vi "New Format.vi"   [LabVIEW 2010]
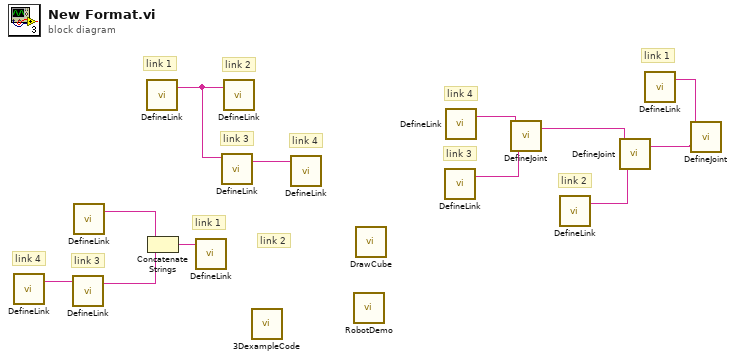
[diagram p0: block diagram]
diagram:
  # "link 1"
  # "link 2"
  # "link 3"
  # "link 4"
  # "link 2"
  # "link 3"
  # "link 4"
  # "link 1"
  # "link 4"
  # "link 3"
  # "link 2"
  # "link 1"
  n1 = call "DefineLink.vi"() -> ("String 2"=w10:string)  [unwired: 4 in]
  n2 = call "DefineLink.vi"("String"=w10) -> ("String 2"=w8:string)  [unwired: 3 in]
  n3 = call "DefineLink.vi"() -> ("String 2"=w9:string)  [unwired: 4 in]
  n4 = call "DefineLink.vi"() -> ("String 2"=w12:string)  [unwired: 4 in]
  n5 = Concatenate Strings(w9, w8) -> (w7:string)
  n6 = call "DefineLink.vi"("String"=w7) -> ()  [unwired: 3 in, 1 out]
  n7 = call "DefineLink.vi"("String"=w12) -> ("String 2"=w11:string)  [unwired: 3 in]
  n8 = call "DefineLink.vi"("String"=w12) -> ()  [unwired: 3 in, 1 out]
  n9 = call "3DexampleCode.vi"() -> ()  [unwired: 12 in]
  n10 = call "DefineLink.vi"("String"=w11) -> ()  [unwired: 3 in, 1 out]
  n11 = call "RobotDemo.vi"() -> ()  [unwired: 12 in]
  n12 = call "DrawCube.vi"() -> ()  [unwired: 6 in, 2 out]
  n13 = call "DefineLink.vi"() -> ("String 2"=w5:string)  [unwired: 4 in]
  n14 = call "DefineLink.vi"() -> ("String 2"=w6:string)  [unwired: 4 in]
  n15 = call "DefineJoint.vi"("String 2"=w5, "String"=w6) -> ("String 3"=w4:string)  [unwired: 2 in]
  n16 = call "DefineLink.vi"() -> ("String 2"=w3:string)  [unwired: 4 in]
  n17 = call "DefineJoint.vi"("String 2"=w3, "String"=w4) -> ("String 3"=w1:string)  [unwired: 2 in]
  n18 = call "DefineLink.vi"() -> ("String 2"=w2:string)  [unwired: 4 in]
  n19 = call "DefineJoint.vi"("String 2"=w1, "String"=w2) -> ()  [unwired: 2 in, 1 out]
